vi "TH_Globals.vi"() -> ()   [LabVIEW 2014]
panel:
  in  "24tim PlotTime":dbl format="%.1f"
  in  "StartTime":dbl format="%.1f"
  out "NewValues":bool[](array[boolean])
  in  "FirstLoopRun":bool=TRUE
  out "Curr_Humidity":dbl[](array[numeric]) format="%.2f"
  out "Curr_Temperature":dbl[](array[numeric]) format="%.2f"
  in  "ExitProgram":bool
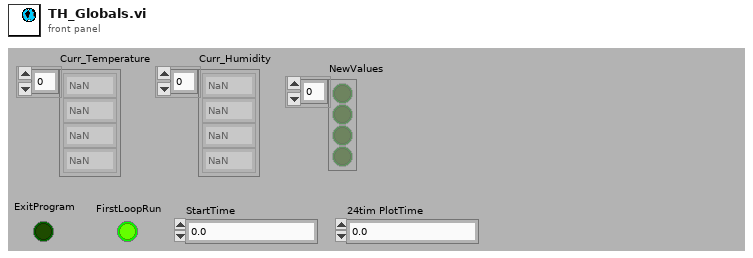
[diagram p1: front panel]
diagram:
